vi "AUTOFLIM_Move_Mirror.vi"(8 "error in (no error)":errorcluster, 9 "Window Cluster":T1, 10 "MG17 Button":enum16{"Position 1", "Position 2"}(ring), 11 "MG17 Cluster":T2) -> (0 "error out":errorcluster)   [LabVIEW 2023]
uses:
  <vilib>/Utility/miscctls.llb/LVPositionTypeDef.ctl
  User32.dll
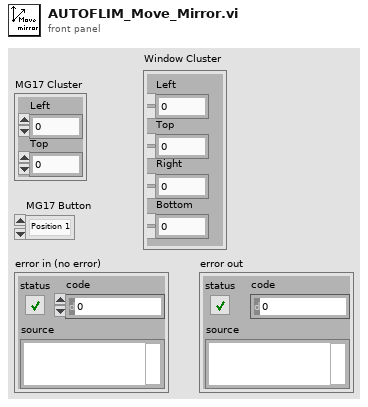
[diagram p1: front panel]
types:
  T1 = cluster{"Left":i32, "Top":i32, "Right":i32, "Bottom":i32}
  T2 = typedef "LVPositionTypeDef.ctl" = cluster{"Left":i32, "Top":i32}
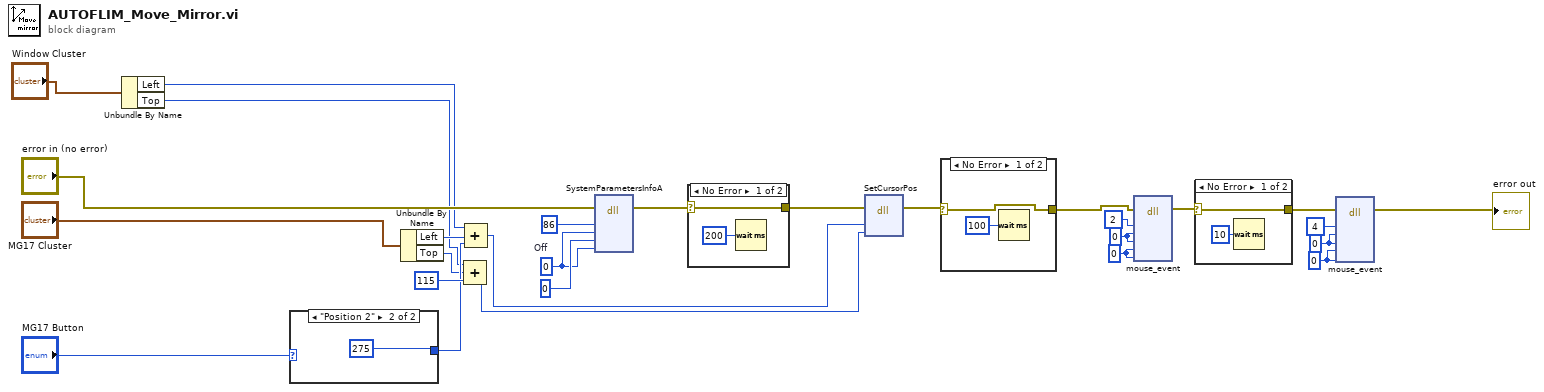
[diagram p0: block diagram]
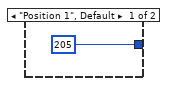
[diagram p3: hidden frame]
diagram:
  w8 = 0 ("dwExtraInfo")
  w7 = u32 0 ("dwExtraInfo")
  w9 = 0 ("dwExtraInfo")
  w10 = u32 0 ("dwExtraInfo")
  w12 = u32 0  # Off
  n1 = Unbundle By Name("Window Cluster") -> ("Left"=w5:i32, "Top"=w4:i32)
  n2 = case shown="\"Position 2\"" "MG17 Button" {
    tunnel: [205 275] -> w25
    frame "Position 1", Default {
    }
    frame "Position 2" {
    }
  }
  n3 = Unbundle By Name("MG17 Cluster") -> ("Left"=w21:i32, "Top"=w20:i32)
  n4 = Compound Arithmetic op=ADD(w4, w20, 115 ("y")) -> (w23:i32)
  n5 = Compound Arithmetic op=ADD(w5, w21, w25) -> (w22:i32)
  n6 = dll-call lib="user32.dll" fn="SystemParametersInfoA" label="Terminate power-off mode"(error in="error in (no error)", "uiAction"=u32 86 ("SPI_GETPOWEROFFACTIVE"), "uiParam"=w12, "pvParam"=0, "fWinIni"=w12) -> (error out=w15:errorcluster)  [unwired: 7 in, 1 out]
  n7 = case shown="No Error" w15 {
    selector: w15 -> [w31 w33]
    tunnel: [w31 w33] -> w16
    frame No Error {
      n8 = Wait (ms)(milliseconds to wait=u32 200) -> ()  [unwired: 1 out]
    }
    frame Error {
    }
  }
  n9 = dll-call lib="user32.dll" fn="SetCursorPos" label="Move mouse"(error in=w16, "dx"=w22, "dy"=w23) -> (error out=w2:errorcluster)  [unwired: 5 in, 1 out]
  n10 = case shown="No Error" w2 {
    selector: w2 -> [w34 w36]
    tunnel: [w34 w36] -> w1
    frame No Error {
      n11 = Wait (ms)(milliseconds to wait=u32 100) -> ()  [unwired: 1 out]
    }
    frame Error {
    }
  }
  n12 = dll-call lib="user32.dll" fn="mouse_event" label="Click"(error in=w1, "dwFlags"=2, "dx"=w9, "dy"=w9, "dwData"=w10, "dwExtraInfo"=w10) -> (error out=w17:errorcluster)  [unwired: 8 in, 1 out]
  n13 = case shown="No Error" w17 {
    selector: w17 -> [w37 w39]
    tunnel: [w37 w39] -> w18
    frame No Error {
      n14 = Wait (ms)(milliseconds to wait=u32 10) -> ()  [unwired: 1 out]
    }
    frame Error {
    }
  }
  n15 = dll-call lib="user32.dll" fn="mouse_event" label="Release"(error in=w18, "dwFlags"=4, "dx"=w8, "dy"=w8, "dwData"=w7, "dwExtraInfo"=w7) -> (error out=→"error out":errorcluster)  [unwired: 8 in, 1 out]
